vi "BeamSteering - Copy.vi"() -> ()   [LabVIEW 2015]
uses:
  <vilib>/Utility/file.llb/Read Delimited Spreadsheet (I64).vi
panel:
  in  "Run":bool=TRUE
  in  "Angle":dbl min=-80.0 max=80.0 step=2.5
  in  "Calibration data path":path=path "C:/Users/zpeng/OneDrive - Texas Tech University/Desktop/BeamSteering/voltages"
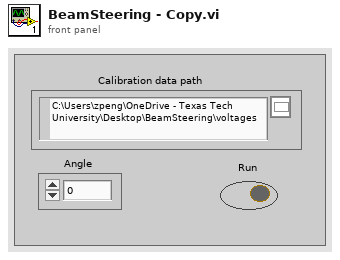
[diagram p1: front panel]
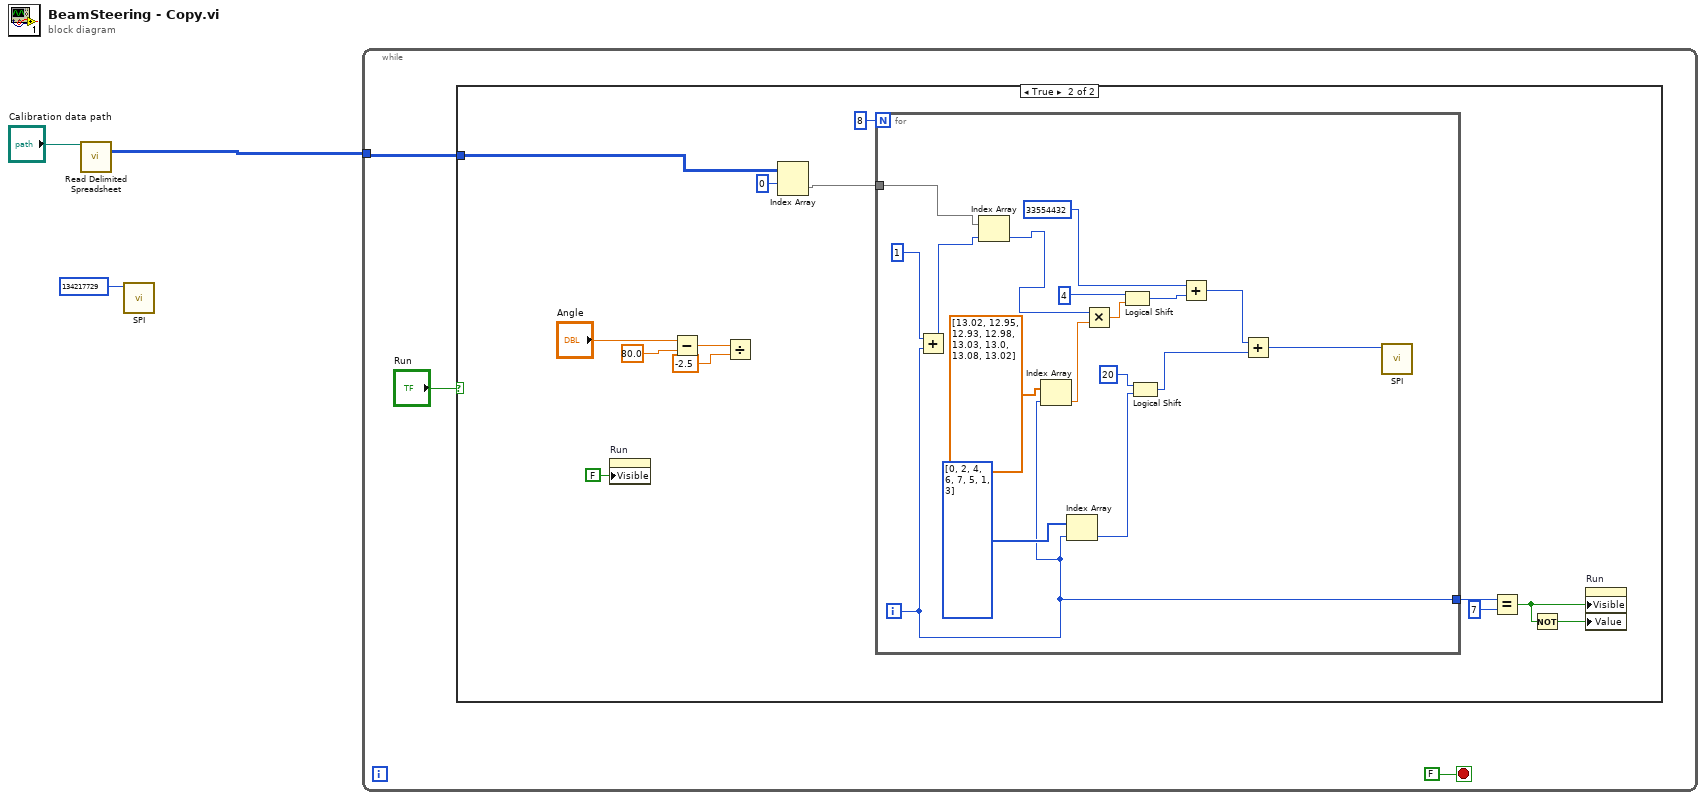
[diagram p0: block diagram]
diagram:
  n1 = call-poly <vilib>:"Read Delimited Spreadsheet.vi"("file path (dialog if empty)"="Calibration data path") -> ("all rows"=w2:i64[][])  [unwired: 9 in, 5 out]
  n2 = call "SPI.vi"("data"=u32 134217729) -> ()  [unwired: 11 in]
  n3 = while {
    tunnel: w2 -> [w6]
    stop <- FALSE stop-if-true
    n4 = case shown="True" "Run" {
      tunnel: w6 -> [_ w14]
      frame False {
      }
      frame True {
        n5 = property on="Run" class="Bool (strict)"("Visible"=FALSE) -> ()  [unwired: 2 in, 2 out]
        n6 = Subtract(x="Angle", y=80.0) -> (x-y=w16:dbl)
        n7 = Divide(x=w16, y=-2.5) -> ()  [unwired: 1 out]
        n8 = Index Array(array=w14, index (row)=0) -> (element=w13:i64[])  [unwired: 1 in]
        n9 = for {
          N: 8 -> [_]
          tunnel: w13 -> [w26]
          tunnel: [w20] -> w12
          i -> [w20]
          n10 = Add(x=1 ("length"), y=w20) -> (x+y=w25:i32)
          n11 = Index Array(array=w26, index=w25) -> (element=w24:i64)
          n12 = Index Array(array=dbl[] [13.02, 12.95, 12.93, 12.98, 13.03, 13.0, 13.08, 13.02] ("y"), index=w20) -> (element=w21:dbl)
          n13 = Index Array(array=i32[] [0, 2, 4, 6, 7, 5, 1, 3], index=w20) -> (element=w23:i32)
          n14 = Multiply(x=w24, y=w21) -> (x*y=w30:dbl)
          n15 = Logical Shift(y=u32 4 ("x"), x=w30) -> (x << y=w35:u32)
          n16 = Logical Shift(y=u32 20 ("x"), x=w23) -> (x << y=w33:i32)
          n17 = Add(x=u32 33554432 ("y"), y=w35) -> (x+y=w34:u32)
          n18 = Add(x=w34, y=w33) -> (x+y=w32:u32)
          n19 = call "SPI.vi"("data"=w32) -> ()  [unwired: 11 in]
        }
        n20 = Equal?(x=w12, y=7) -> (x = y?=w8:bool)
        n21 = Not(x=w8) -> (.not. x?=w9:bool)
        n22 = property on="Run" class="Bool (strict)"("Visible"=w8, "Value"=w9) -> ()  [unwired: 2 in, 2 out]
      }
    }
  }
